vi "SubMatrixVg2.vi"(0 "VgCluster":T1={"Target Voltage, V"=1.0, "Sweep rate, V/min"=1.0, "Time btw \npoints, sec"=1.0, "points at each Vg"=1, "Set compliance limit, mkA"=0.05} {"Set compliance limit, mkA" min=0.0 max=1.0 step=0.01 format="%.3f"; "Time btw \npoints, sec" format="%.2f"; "Sweep rate, V/min" min=0.0 max=1.0 step=0.01 format="%.4f"; "Target Voltage, V" min=-4.0 max=4.0 step=0.1 format="%.4f"}, 1 "Instruments":T3={"Oscillator"=TRUE, "Addr 1 lock-in"=TRUE, "Addr 1 lock-in oop"=TRUE, "Addr 2 lock-in"=FALSE, "Addr 2 lock-in oop"=FALSE, "Addr 3 lock-in"=FALSE, "Addr 3 lock-in oop"=FALSE, "Voltage (Vk1)"=FALSE, "Current (Ik1)"=TRUE, "Voltage (Vk2)"=FALSE, "Current (Ik2)"=FALSE, "Voltage (Vk3)"=FALSE, "Current (Ik3)"=FALSE, "Channel 1 (Vnano1)  "=FALSE, "Channel 2 (Vnano1b)"=FALSE, "Channel 1 (Vnano2)   "=FALSE, "Channel 2 (Vnano2b)"=FALSE, "Thermometer 1 (T1)"=TRUE, "Magnetic Field (B)"=TRUE, "Capacitance (C) and Loss (L)"=FALSE}, 2 "Settings":T2={"Ring 3"=1, "Ring 2"=4, "Fixed Current mkA"=0.5, "If yes, the current is:"=enum."Radio Selection 1", "Ressitance measurements?"=TRUE, "Commute DC current?"=FALSE} {"Ring 3" items=["1 kOhm", "10 kOhm", "100 kOhm", "1 Mohm", "10 mOhm"]; "Ring 2" items=["1 kOhm", "10 kOhm", "100 kOhm", "1 Mohm", "10 MOhm"]}, 3 "Custom Folder":string, 4 "Time Stamp":timestamp) -> ()   [LabVIEW 2017]
uses:
  <vilib>/Utility/file.llb/Write To Spreadsheet File (DBL).vi
panel:
  out "Vk2ini":dbl
  out "Current":dbl
  out "Comments":string[](array[string])
  out "ArrayBoolian":bool[][](array[boolean])
  out "Delib Time delay":i32
  out "XY Graph":cluster{dbl[], dbl[]}(graph)={[1.0, 0.8, 0.6000000000000001, 0.4000000000000001, 0.20000000000000007, 5.551115123125783e-17, -0.19999999999999996, -0.39999999999999997, -0.6, -0.8, -1.0], [0.03352775, 0.056811, 0.03911575, 0.04330675, -0.02468015, 0.011641600000000002, 0.10151450000000001, 0.12386675000000001, 0.08288825000000001, -0.00186266, -0.038650000000000004]}
  out "array for data":dbl[](array[numeric])
  in  "Ring":u16(ring) caption="Y-axis:" items=["Vg"]
  out "Data file:":path
  in  "error in (no error)":errorcluster
  # "Lock-in Amplifiers"
  # "Temperature"
  # "SourceMeters"
  # "Nanovoltmeters"
  # "Main"
  # "(not recommended, too slow)"
  # "Magnetic Field"
  # "Capacitance & Loss"
  # "(not recommended, too slow)"
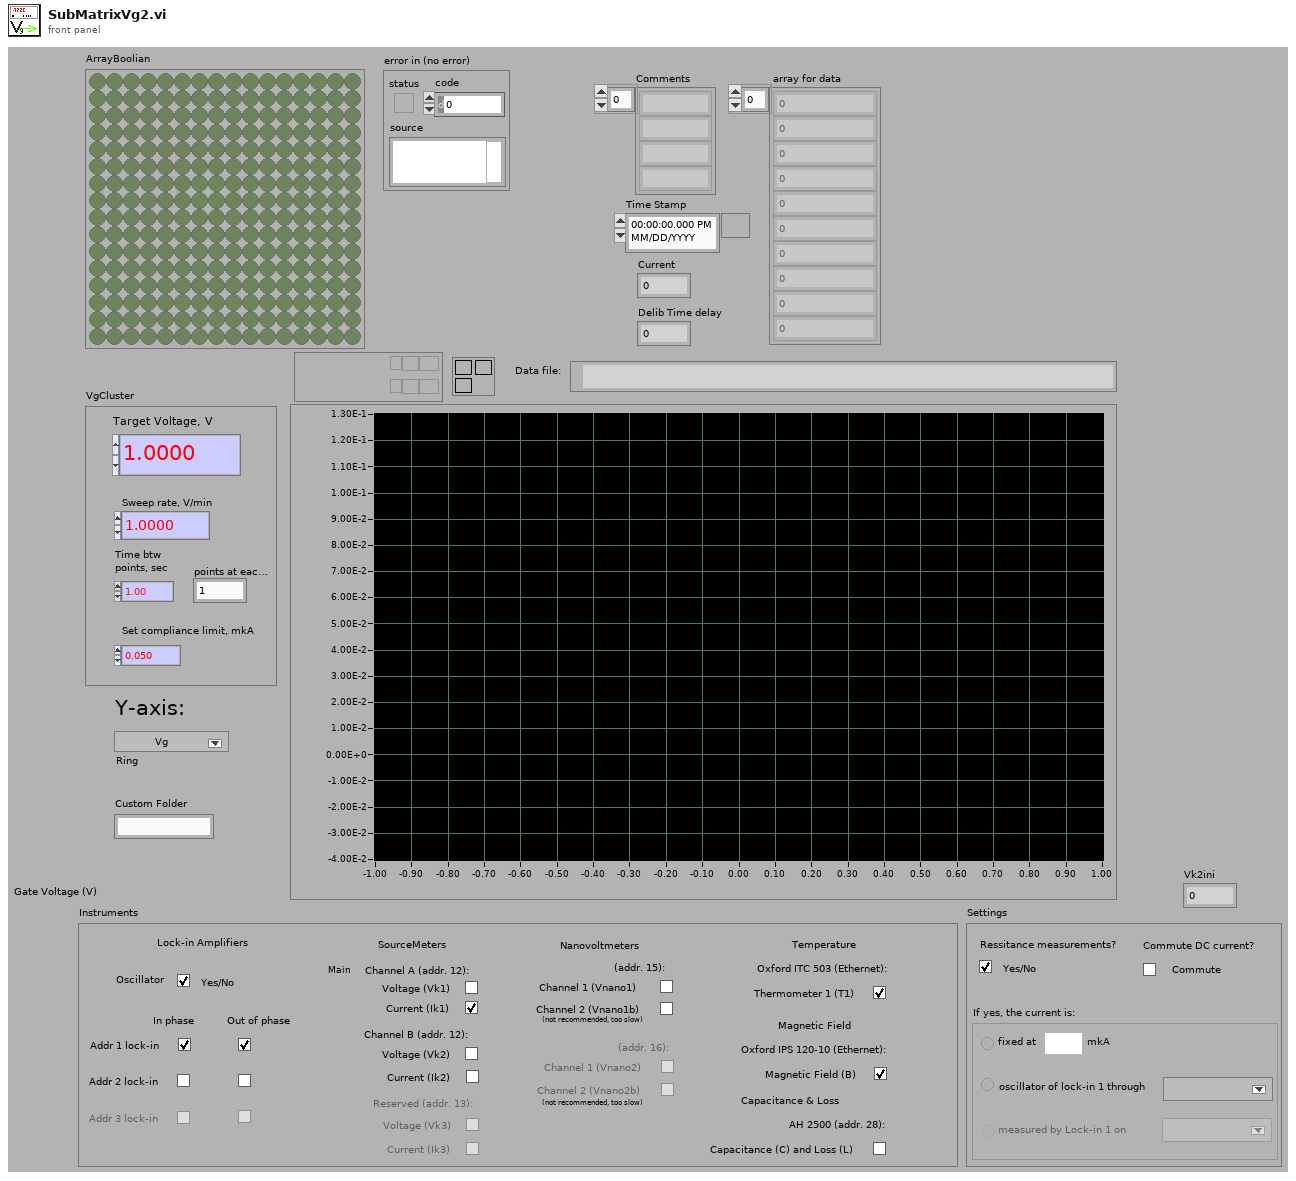
[diagram p1: front panel]
types:
  T1 = cluster{"Target Voltage, V":dbl, "Sweep rate, V/min":dbl, "Time btw \npoints, sec":dbl, "points at each Vg":i32, "Set compliance limit, mkA":dbl}
  T2 = cluster{"Ring 3":u16, "Ring 2":u16, "Fixed Current mkA":dbl, "If yes, the current is:":enum32{"Radio Selection 1", "Radio Selection 2", "Radio Selection 3"}, "Ressitance measurements?":bool, "Commute DC current?":bool}
  T3 = cluster{"Oscillator":bool, "Addr 1 lock-in":bool, "Addr 1 lock-in oop":bool, "Addr 2 lock-in":bool, "Addr 2 lock-in oop":bool, "Addr 3 lock-in":bool, "Addr 3 lock-in oop":bool, "Voltage (Vk1)":bool, "Current (Ik1)":bool, "Voltage (Vk2)":bool, "Current (Ik2)":bool, "Voltage (Vk3)":bool, "Current (Ik3)":bool, "Channel 1 (Vnano1)  ":bool, "Channel 2 (Vnano1b)":bool, "Channel 1 (Vnano2)   ":bool, "Channel 2 (Vnano2b)":bool, "Thermometer 1 (T1)":bool, "Magnetic Field (B)":bool, "Capacitance (C) and Loss (L)":bool}
  T4 = enum32{"Radio Selection 1", "Radio Selection 2", "Radio Selection 3"}
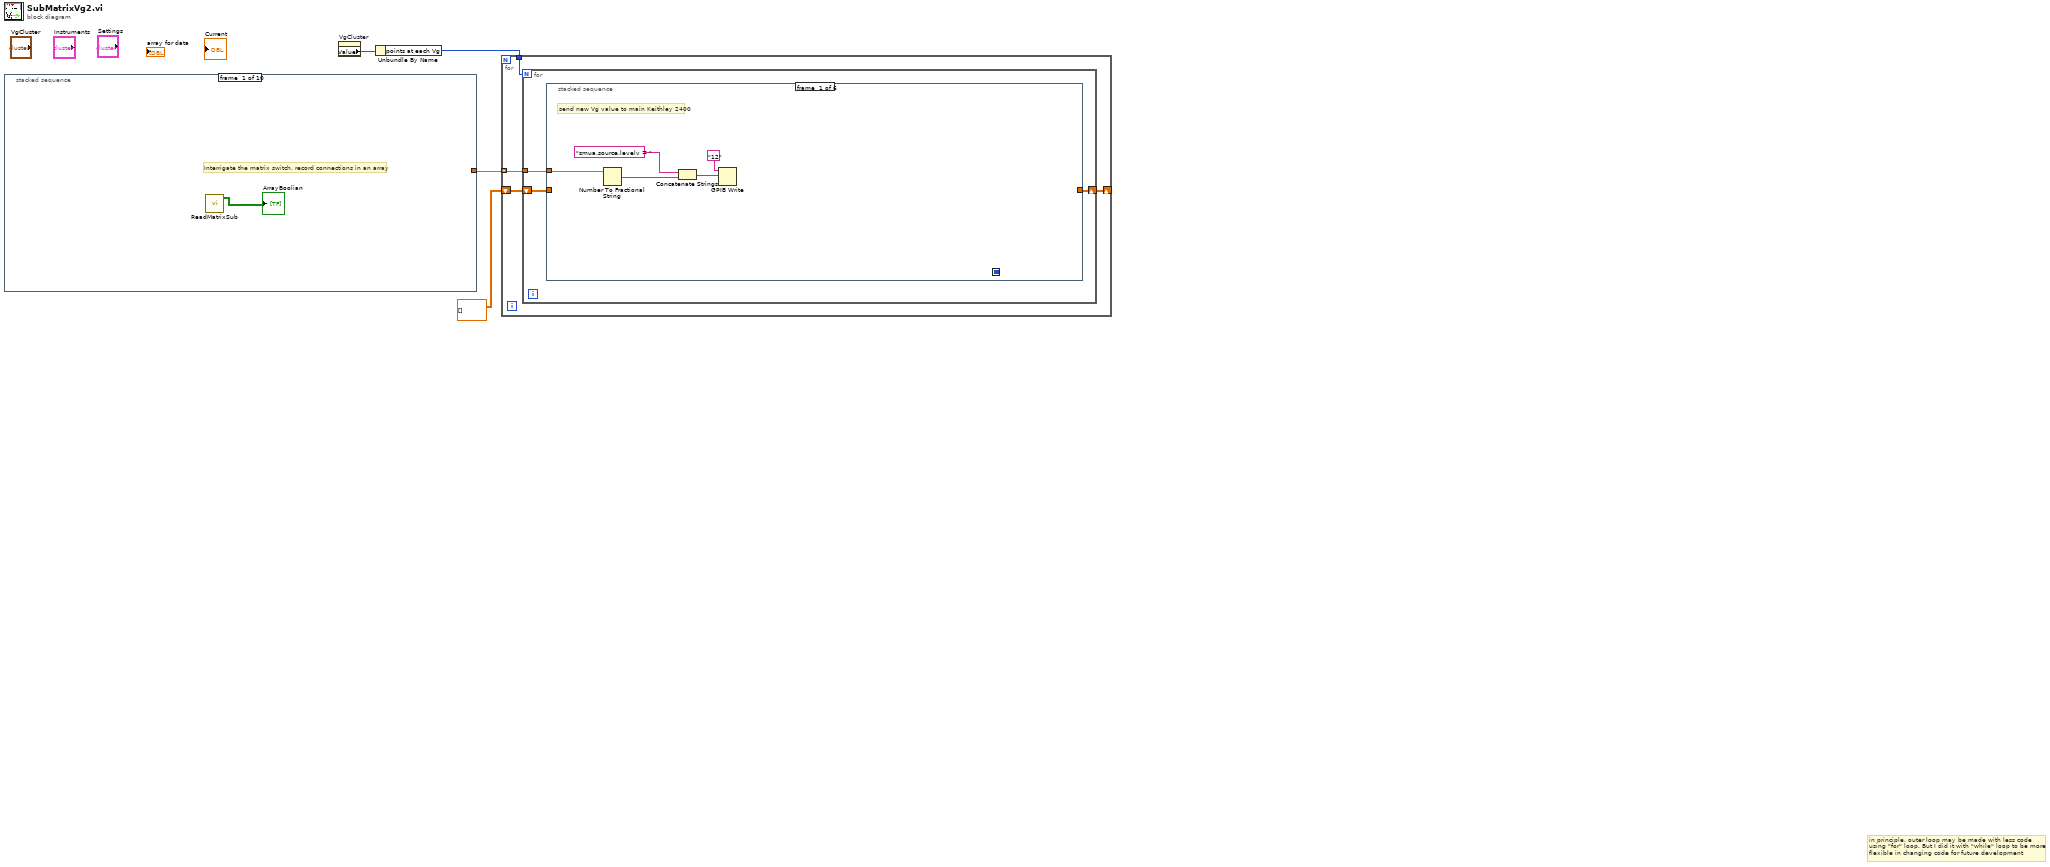
[diagram p0: block diagram]
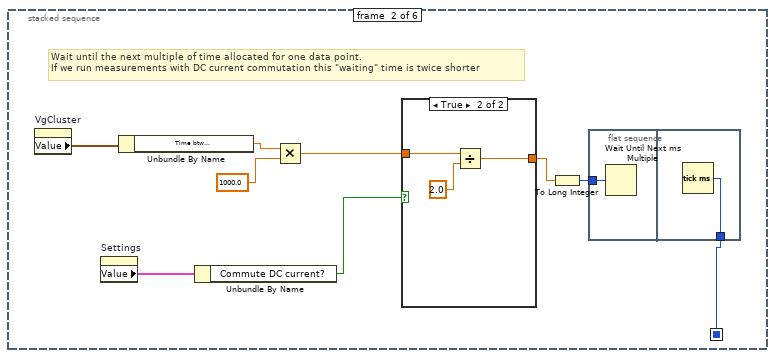
[diagram p2: hidden frame]
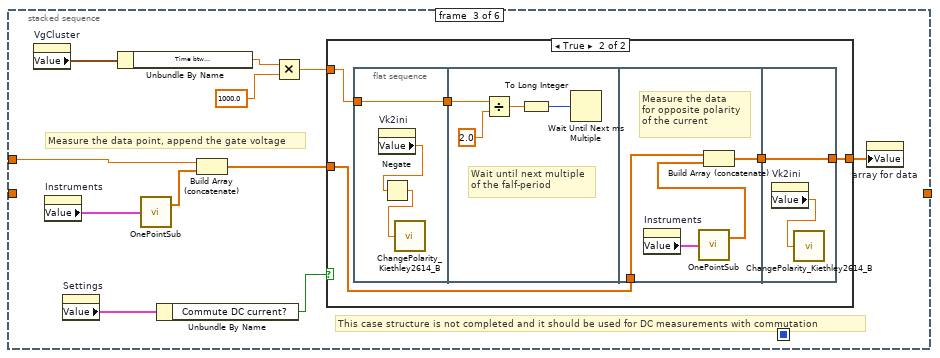
[diagram p4: hidden frame]
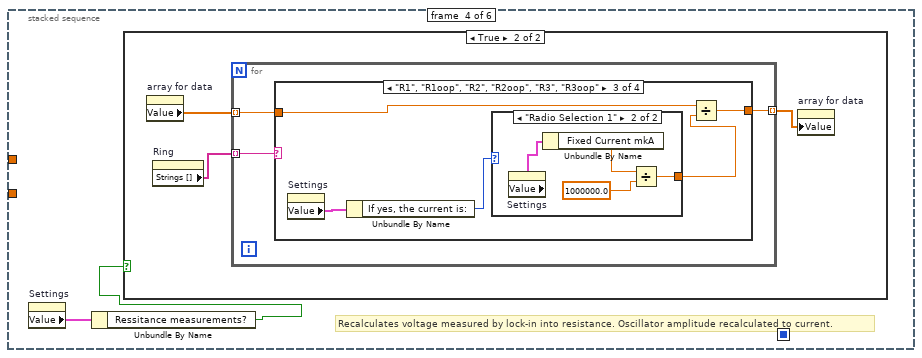
[diagram p6: hidden frame]
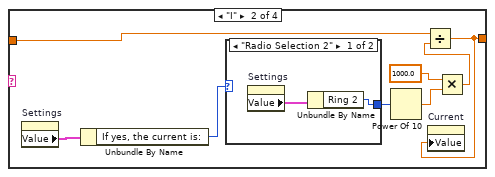
[diagram p9: hidden frame]
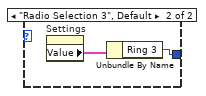
[diagram p10: hidden frame]
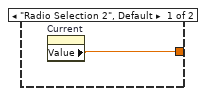
[diagram p11: hidden frame]
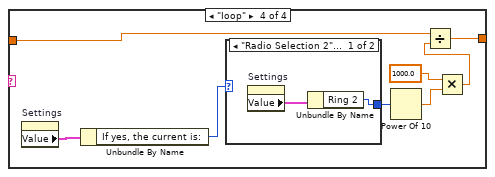
[diagram p12: hidden frame]
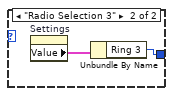
[diagram p13: hidden frame]
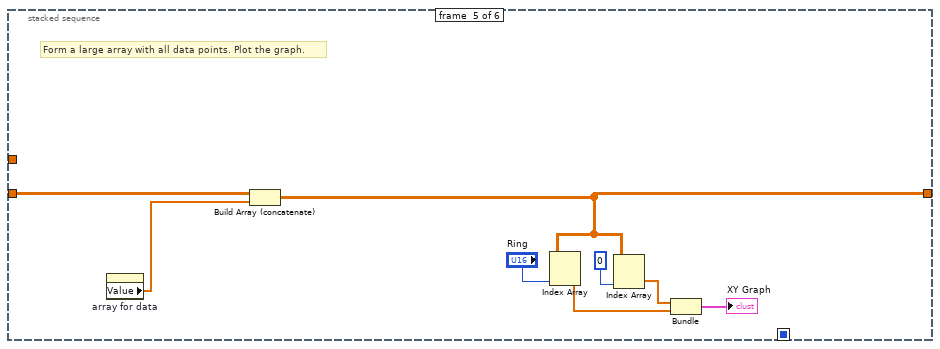
[diagram p14: hidden frame]
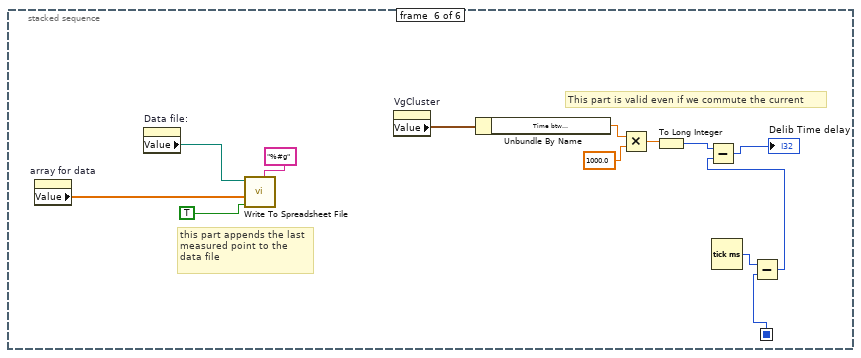
[diagram p15: hidden frame]
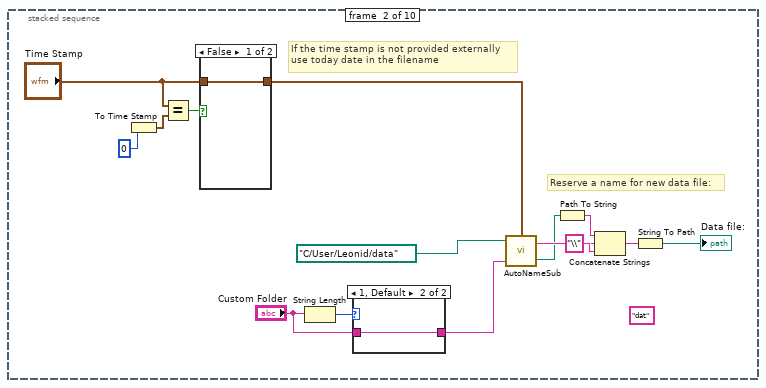
[diagram p16: hidden frame]
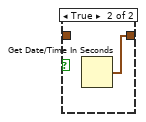
[diagram p17: hidden frame]
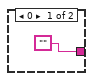
[diagram p18: hidden frame]
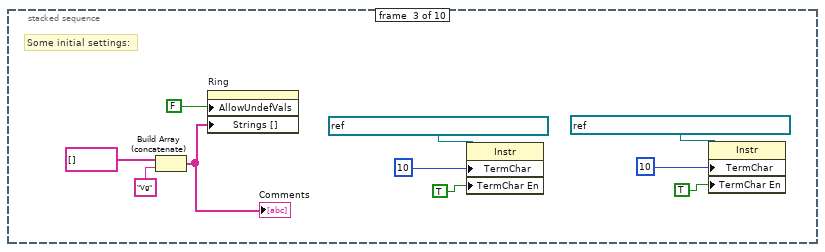
[diagram p19: hidden frame]
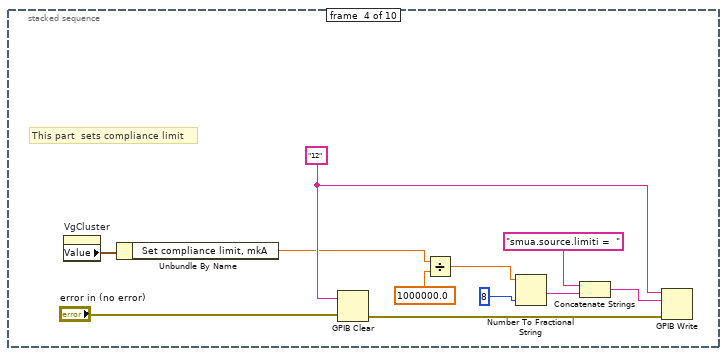
[diagram p20: hidden frame]
diagram:
  # "in principle, outer loop may be made with less code\nusing \"for\" loop. But I did it with \"while\" loop to be more \nflexible in changing code for future development"
  n1 = stacked-sequence {
    tunnel: [_ _ _ _ _ _ _ _ _ w128] -> w4
    frame #0 {
      # "Interrigate the matrix switch, record connections in an array"
      n2 = call "ReadMatrixSub.vi"() -> ("Array"=→"ArrayBoolian":bool[][])  [unwired: 9 in, 2 out]
    }
    frame #1 {
      (unwired) "dat"
      # "If the time stamp is not provided externally\nuse today date in the filename"
      # "Reserve a name for new data file:"
      n3 = To Time Stamp(1:0) -> (0:w9:timestamp)
      n4 = Equal?(x="Time Stamp", y=w9) -> (x = y?=w8:bool)
      n5 = case shown="False" w8 {
        tunnel: "Time Stamp" -> [w21 _]
        tunnel: [w21 w22] -> w6
        frame False {
        }
        frame True {
          n6 = Get Date/Time In Seconds() -> (seconds since 1Jan1904=w22:timestamp)
        }
      }
      n7 = String Length(string="Custom Folder") -> (length=w13:i32)
      n8 = case shown="1, Default" w13 {
        tunnel: "Custom Folder" -> [_ w24]
        tunnel: ["" w24] -> w11
        frame 0 {
        }
        frame 1, Default {
        }
      }
      n9 = call "AutoNameSub.vi"("Time Stamp"=w6, "Custom Folder"=w11, "User Data Folder"=path "C:/User/Leonid/data") -> ("created path"=w19:path, "String"=w20:string)  [unwired: 1 in]
      n10 = Path To String(path=w19) -> (string=w14:string)
      n11 = Concatenate Strings(w14, "\\", w20) -> (w16:string)
      n12 = String To Path(string=w16) -> (path=→"Data file:":path)
    }
    frame #2 {
      # "Some initial settings:"
      n13 = Build Array (concatenate)(string[] [], "Vg") -> (w25:string[])
      "Comments" <- w25
      n14 = property on="Ring" class="Ring (strict)"("AllowUndefVals"=FALSE, "Strings []"=w25) -> ()  [unwired: 2 in, 2 out]
      n15 = property class="Instr"(reference=refnum<visa-resource-name> "TCPIP0::192.168.128.3::7020::SOCKET" ("VISA resource name"), "TermChar"=10, "TermChar En"=TRUE) -> ()  [unwired: 1 in, 2 out]
      n16 = property class="Instr"(reference=refnum<visa-resource-name> "TCPIP0::192.168.128.2::7020::SOCKET" ("VISA resource name"), "TermChar"=10, "TermChar En"=TRUE) -> ()  [unwired: 1 in, 2 out]
    }
    frame #3 {
      w38 = "12"
      # "This part  sets compliance limit"
      n17 = property on="VgCluster" class="Clust (strict)"() -> ("Value"=w36:T1)  [unwired: 2 in, 2 out]
      n18 = Unbundle By Name(w36) -> ("Set compliance limit, mkA"=w35:dbl)
      n19 = GPIB Clear(2:"error in (no error)", 3:w38) -> (0:w39:errorcluster)  [unwired: 1 out]
      n20 = Divide(x=w35, y=1000000.0) -> (x/y=w44:dbl)
      n21 = Number To Fractional String(number=w44, precision (6)=i16 8) -> (F-format string=w41:string)  [unwired: 2 in]
      n22 = Concatenate Strings("smua.source.limiti =  " ("data"), w41) -> (w40:string)
      n23 = GPIB Write(0:w38, 1:w40, 3:w39) -> ()  [unwired: 2 in, 2 out]
    }
    frame #4 {
      # "List of measured parameters obtained as \na text array and \"fed\" to a ring selector"
      # "When current is commutated every data point is measured twice (for both polarities of DC current). Names \nof parameters measured for negative polarity will start with lower case \"c\" (for \"commutated\")"
      # "Measurement of one data point (only to get the names of the parameters to be recorded)"
      n24 = property on="Settings" class="Clust (strict)"() -> ("Value"=w52:T2)  [unwired: 2 in, 2 out]
      n25 = property on="Instruments" class="Clust (strict)"() -> ("Value"=w50:T3)  [unwired: 2 in, 2 out]
      n26 = Unbundle By Name(w52) -> ("Commute DC current?"=w53:bool)
      n27 = call "OnePointSub.vi"("cluster"=w50) -> ("TextArray"=w51:string[], "Array"=w46:dbl[])  [unwired: 2 in]
      n28 = case shown="True" w53 {
        tunnel: w51 -> [w55 w64]
        tunnel: [w57 w64] -> w49
        tunnel: w46 -> [w54 _]
        frame True {
          (unwired) 1
          n29 = for {
            tunnel: w55 -> [w59] mode=indexing
            tunnel: w54 -> [w58] mode=indexing
            n30 = case shown="Default" w59 {
              tunnel: w58 -> [w60 _]
              frame "Vk2" {
                "Vk2ini" <- w60
              }
              frame Default {
              }
            }
          }
          n31 = for {
            tunnel: [w63] -> w56 mode=indexing
            tunnel: w55 -> [w61] mode=indexing
            n32 = Concatenate Strings("c", w61) -> (w63:string)
          }
          n33 = Build Array (concatenate)(w55, w56) -> (w57:string[])
        }
        frame False {
        }
      }
      n34 = Build Array (concatenate)("Vg", w49) -> (w47:string[])
      n35 = property on="Ring" class="Ring (strict)"("Strings []"=w47) -> ()  [unwired: 2 in, 2 out]
    }
    frame #5 {
      # "If resistance is not something that we are interested in, then replace \"R\" with \"V\" in all strings"
      n36 = property on="Settings" class="Clust (strict)"() -> ("Value"=w65:T2)  [unwired: 2 in, 2 out]
      n37 = Unbundle By Name(w65) -> ("Ressitance measurements?"=w66:bool)
      n38 = case shown="False" w66 {
        frame True {
        }
        frame False {
          n39 = property on="Ring" class="Ring (strict)"() -> ("Strings []"=w68:string[])  [unwired: 2 in, 2 out]
          n40 = for {
            tunnel: w68 -> [w71] mode=indexing
            tunnel: [w69] -> w67 mode=indexing
            n41 = String Subset(string=w71, length (rest)=1) -> (substring=w73:string)  [unwired: 1 in]
            n42 = Equal?(x=w73, y="R") -> (x = y?=w72:bool)
            n43 = case shown="True" w72 {
              tunnel: w71 -> [w75 w79]
              tunnel: [w75 w76] -> w69
              frame False {
              }
              frame True {
                n44 = Replace Substring(2:1, 4:"V", 5:w79) -> (1:w76:string)  [unwired: 1 in, 1 out]
              }
            }
          }
          n45 = property on="Ring" class="Ring (strict)"("Strings []"=w67) -> ()  [unwired: 2 in, 2 out]
        }
      }
    }
    frame #6 {
      # "This part makes comment line for the \ndata file. Comments are very useful for\ndouble checking that connections are \ncorrect when the data file is opened\nin Origin."
      # "Check how the oscillator is wired to the matrix switch and record connection as a comment"
      n46 = property on="Instruments" class="Clust (strict)"() -> ("Value"=w82:T3)  [unwired: 2 in, 2 out]
      n47 = property on="Comments" class="Arr (strict)"() -> ("Value"=w81:string[])  [unwired: 2 in, 2 out]
      n48 = Unbundle By Name(w82) -> ("Oscillator"=w83:bool)
      n49 = case shown="True" w83 {
        tunnel: [w84 w87] -> w80
        tunnel: w81 -> [w84 w86]
        frame False {
          # "we are not measuring oscillator from\nlock-in (address 1)"
        }
        frame True {
          (unwired) "I"
          # "This subVI takes the matrix column # (instrument\nconnection point) as an argument and finds the raw\n# (contact) to which the instrument is connected"
          # "we are  measuring oscillator"
          n50 = property on="ArrayBoolian" class="Arr (strict)"() -> ("Value"=w90:bool[][])  [unwired: 2 in, 2 out]
          n51 = GPIB Clear(3:"1") -> ()  [unwired: 1 in, 2 out]
          n52 = call "FindInstrConnect.vi"("Column #"=1, "ArrayBoolian"=w90) -> ("String"=w91:string)  [unwired: 1 in, 2 out]
          n53 = call "FindInstrConnect.vi"("Column #"=0, "ArrayBoolian"=w90) -> ("String"=w88:string)  [unwired: 1 in, 2 out]
          n54 = Concatenate Strings(w88, "-", w91) -> (w85:string)
          n55 = Build Array (concatenate)(w86, w85) -> (w87:string[])
        }
      }
      n56 = property on="Comments" class="Arr (strict)"("Value"=w80) -> ()  [unwired: 2 in, 2 out]
    }
    frame #7 {
      # "Check how the input of Lock-in 1 is wired the the matrix switch and record connection as a comment"
      n57 = property on="Instruments" class="Clust (strict)"() -> ("Value"=w97:T3)  [unwired: 2 in, 2 out]
      n58 = property on="Comments" class="Arr (strict)"() -> ("Value"=w96:string[])  [unwired: 2 in, 2 out]
      n59 = Unbundle By Name(w97) -> ("Addr 1 lock-in"=w98:bool)
      n60 = case shown="True" w98 {
        tunnel: [w99 w102] -> w95
        tunnel: w96 -> [w99 w101]
        frame False {
          # "we are not measuring oscillator from\nlock-in (address 1)"
        }
        frame True {
          (unwired) "I"
          # "This subVI takes the matrix column # (instrument\nconnection point) as an argument and finds the raw\n# (contact) to which the instrument is connected"
          # "we are  measuring Lock-In 1"
          n61 = property on="ArrayBoolian" class="Arr (strict)"() -> ("Value"=w105:bool[][])  [unwired: 2 in, 2 out]
          n62 = GPIB Clear(3:"1") -> ()  [unwired: 1 in, 2 out]
          n63 = call "FindInstrConnect.vi"("Column #"=3, "ArrayBoolian"=w105) -> ("String"=w106:string)  [unwired: 1 in, 2 out]
          n64 = call "FindInstrConnect.vi"("Column #"=2, "ArrayBoolian"=w105) -> ("String"=w103:string)  [unwired: 1 in, 2 out]
          n65 = Concatenate Strings(w103, "-", w106) -> (w100:string)
          n66 = Build Array (concatenate)(w101, w100) -> (w102:string[])
        }
      }
      n67 = property on="Comments" class="Arr (strict)"("Value"=w95) -> ()  [unwired: 2 in, 2 out]
    }
    frame #8 {
      w118 = "\r"
      w117 = "\n"
      # "Both lines are recorded into\nthe data file."
      # "This part converts string array with the names of measured parameters into the line of text separated by TABs. The resulting string is\nrecorded as the first line of the data file. The second line is comments with information about conections of the instruments to particular contacts."
      n68 = property on="Ring" class="Ring (strict)"() -> ("Strings []"=w111:string[])  [unwired: 2 in, 2 out]
      n69 = property on="Comments" class="Arr (strict)"() -> ("Value"=w116:string[])  [unwired: 2 in, 2 out]
      n70 = for {
        tunnel: w111 -> [w126] mode=indexing
        shift-right: [w124] -> w114
        shift-left: "" -> [w125]
        n71 = Concatenate Strings(w125, w126, "\t") -> (w124:string)
      }
      n72 = for {
        tunnel: w116 -> [w122] mode=indexing
        shift-right: [w120] -> w119
        shift-left: "" -> [w121]
        n73 = Concatenate Strings(w121, w122, "\t") -> (w120:string)
      }
      n74 = Concatenate Strings(w114, w118, w117, w118, w117, w119, w118, w117) -> (w112:string)
      n75 = property on="Data file:" class="Path"() -> ("Value"=w110:path)  [unwired: 2 in, 2 out]
      n76 = Write to Text File(file (use dialog)=w110, text=w112) -> ()  [unwired: 2 in, 3 out]
    }
    frame #9 {
      w142 = "12"
      # "Then the table is made with all values\nof the gate voltage to be measured"
      # "rounding to 0.1 V"
      # "This part reads the output voltage on channel A of the main Keithly 2614B \n(address 12)"
      n77 = property on="VgCluster" class="Clust (strict)"() -> ("Value"=w136:T1)  [unwired: 2 in, 2 out]
      n78 = Unbundle By Name(w136) -> ("Target Voltage, V"=w130:dbl, "Sweep rate, V/min"=w135:dbl, "Time btw \npoints, sec"=w134:dbl)
      n79 = GPIB Write(0:w142, 1:"print(smua.measure.v())" ("data")) -> (6:w145:errorcluster)  [unwired: 3 in, 1 out]
      n80 = GPIB Read(0:w142, 1:200 ("byte count"), 3:w145) -> (5:w137:string)  [unwired: 2 in, 2 out]
      n81 = Fract/Exp String To Number(string=w137) -> (number=w141:dbl)  [unwired: 3 in, 1 out]
      n82 = Multiply(x=w135, y=w134) -> (x*y=w133:dbl)
      n83 = Divide(x=w133, y=60.0) -> (x/y=w129:dbl)
      n84 = Number To Fractional String(number=w141, width (-)=5, precision (6)=1) -> (F-format string=w138:string)  [unwired: 1 in]
      n85 = Fract/Exp String To Number(string=w138) -> (number=w131:dbl)  [unwired: 3 in, 1 out]
      n86 = call "LinTableSubVI.vi"("Step"=w129, "Final"=w130, "Initial"=w131) -> ("Array"=w128:dbl[])  [unwired: 1 in]
    }
  }
  n87 = property on="VgCluster" class="Clust (strict)"() -> ("Value"=w3:T1)  [unwired: 2 in, 2 out]
  n88 = Unbundle By Name(w3) -> ("points at each Vg"=w2:i32)
  n89 = for {
    tunnel: w4 -> [w149] mode=indexing
    tunnel: w2 -> [w148]
    shift-right: [w146] -> _
    shift-left: dbl[][] [] -> [w147]
    n90 = for {
      N: w148 -> [_]
      tunnel: w149 -> [w152]
      shift-right: [w150] -> w146
      shift-left: w147 -> [w151]
      n91 = stacked-sequence {
        seq-local: [_ w158 _ _ _ _] -> [_ _ _ _ _ w261]
        tunnel: w152 -> [w154 _ w175 _ _ _]
        tunnel: w151 -> [_ _ _ _ w248 _]
        tunnel: [_ _ _ _ w246 _] -> w150
        frame #0 {
          # "send new Vg value to main Keithley 2400"
          n92 = Number To Fractional String(number=w154) -> (F-format string=w156:string)  [unwired: 3 in]
          n93 = Concatenate Strings("smua.source.levelv = " ("data"), w156) -> (w155:string)
          n94 = GPIB Write(0:"12", 1:w155) -> ()  [unwired: 3 in, 2 out]
        }
        frame #1 {
          # "Wait until the next multiple of time allocated for one data point.\nIf we run measurements with DC current commutation this \"waiting\" time is twice shorter"
          n95 = property on="VgCluster" class="Clust (strict)"() -> ("Value"=w166:T1)  [unwired: 2 in, 2 out]
          n96 = property on="Settings" class="Clust (strict)"() -> ("Value"=w163:T2)  [unwired: 2 in, 2 out]
          n97 = Unbundle By Name(w166) -> ("Time btw \npoints, sec"=w165:dbl)
          n98 = Unbundle By Name(w163) -> ("Commute DC current?"=w162:bool)
          n99 = Multiply(x=w165, y=1000.0) -> (x*y=w161:dbl)
          n100 = case shown="True" w162 {
            tunnel: w161 -> [w169 w171]
            tunnel: [w169 w170] -> w160
            frame False {
            }
            frame True {
              n101 = Divide(x=w171, y=2.0) -> (x/y=w170:dbl)
            }
          }
          n102 = To Long Integer(number=w160) -> (32bit integer=w159:i32)
          n103 = flat-sequence {
            tunnel: w159 -> [w167]
            tunnel: [w168] -> w158
            frame #0 {
              n104 = Wait Until Next ms Multiple(millisecond multiple=w167) -> ()  [unwired: 1 out]
            }
            frame #1 {
              n105 = Tick Count (ms)() -> (millisecond timer value=w168:u32)
            }
          }
        }
        frame #2 {
          # "This case structure is not completed and it should be used for DC measurements with commutation"
          # "Measure the data point, append the gate voltage"
          n106 = property on="VgCluster" class="Clust (strict)"() -> ("Value"=w183:T1)  [unwired: 2 in, 2 out]
          n107 = property on="Instruments" class="Clust (strict)"() -> ("Value"=w177:T3)  [unwired: 2 in, 2 out]
          n108 = property on="Settings" class="Clust (strict)"() -> ("Value"=w180:T2)  [unwired: 2 in, 2 out]
          n109 = Unbundle By Name(w183) -> ("Time btw \npoints, sec"=w182:dbl)
          n110 = call "OnePointSub.vi"("cluster"=w177) -> ("Array"=w176:dbl[])  [unwired: 2 in, 1 out]
          n111 = Unbundle By Name(w180) -> ("Commute DC current?"=w179:bool)
          n112 = Build Array (concatenate)(w175, w176) -> (w174:dbl[])
          n113 = Multiply(x=w182, y=1000.0) -> (x*y=w178:dbl)
          n114 = case shown="True" w179 {
            tunnel: w178 -> [_ w189]
            tunnel: [w184 w186] -> w173
            tunnel: w174 -> [w184 w187]
            frame False {
            }
            frame True {
              n115 = flat-sequence {
                tunnel: w189 -> [w192]
                tunnel: [w192] -> w188
                tunnel: w188 -> [w195]
                tunnel: w187 -> [w198]
                tunnel: [w197] -> w185
                tunnel: [w202] -> w186
                tunnel: w185 -> [w202]
                frame #0 {
                  n116 = property on="Vk2ini" class="DigNum (strict)"() -> ("Value"=w190:dbl)  [unwired: 2 in, 2 out]
                  n117 = Negate(x=w190) -> (-x=w191:dbl)
                  n118 = call "ChangePolarity_Kiethley2614_B.vi"("Voltage (sourse)"=w191) -> ()  [unwired: 1 in]
                }
                frame #1 {
                  # "Wait until next multiple\nof the falf-period"
                  n119 = Divide(x=w195, y=2.0) -> (x/y=w193:dbl)
                  n120 = To Long Integer(number=w193) -> (32bit integer=w194:i32)
                  n121 = Wait Until Next ms Multiple(millisecond multiple=w194) -> ()  [unwired: 1 out]
                }
                frame #2 {
                  # "Measure the data\nfor opposite polarity\nof the current"
                  n122 = property on="Instruments" class="Clust (strict)"() -> ("Value"=w200:T3)  [unwired: 2 in, 2 out]
                  n123 = call "OnePointSub.vi"("cluster"=w200) -> ("Array"=w199:dbl[])  [unwired: 2 in, 1 out]
                  n124 = Build Array (concatenate)(w198, w199) -> (w197:dbl[])
                }
                frame #3 {
                  n125 = property on="Vk2ini" class="DigNum (strict)"() -> ("Value"=w201:dbl)  [unwired: 2 in, 2 out]
                  n126 = call "ChangePolarity_Kiethley2614_B.vi"("Voltage (sourse)"=w201) -> ()  [unwired: 1 in]
                }
              }
            }
          }
          n127 = property on="array for data" class="Arr (strict)"("Value"=w173) -> ()  [unwired: 2 in, 2 out]
        }
        frame #3 {
          # "Recalculates voltage measured by lock-in into resistance. Oscillator amplitude recalculated to current."
          n128 = property on="Settings" class="Clust (strict)"() -> ("Value"=w204:T2)  [unwired: 2 in, 2 out]
          n129 = Unbundle By Name(w204) -> ("Ressitance measurements?"=w203:bool)
          n130 = case shown="True" w203 {
            frame False {
            }
            frame True {
              n131 = property on="array for data" class="Arr (strict)"() -> ("Value"=w206:dbl[])  [unwired: 2 in, 2 out]
              n132 = property on="Ring" class="Ring (strict)"() -> ("Strings []"=w207:string[])  [unwired: 2 in, 2 out]
              n133 = for {
                tunnel: w207 -> [w210] mode=indexing
                tunnel: w206 -> [w209] mode=indexing
                tunnel: [w208] -> w205 mode=indexing
                n134 = case shown="\"R1\", \"R1oop\", \"R2\", \"R2oop\", \"R3\", \"R3oop\"" w210 {
                  tunnel: w209 -> [w211 w214 w226 w236]
                  tunnel: [w211 w212 w225 w235] -> w208
                  frame "False", Default {
                  }
                  frame "I" {
                    n135 = property on="Settings" class="Clust (strict)"() -> ("Value"=w219:T2)  [unwired: 2 in, 2 out]
                    n136 = Unbundle By Name(w219) -> ("If yes, the current is:"=w218:T4)
                    n137 = case shown="\"Radio Selection 2\"" w218 {
                      tunnel: [w220 w222] -> w213
                      frame "Radio Selection 2" {
                        n138 = property on="Settings" class="Clust (strict)"() -> ("Value"=w221:T2)  [unwired: 2 in, 2 out]
                        n139 = Unbundle By Name(w221) -> ("Ring 2"=w220:u16)
                      }
                      frame "Radio Selection 3", Default {
                        n140 = property on="Settings" class="Clust (strict)"() -> ("Value"=w223:T2)  [unwired: 2 in, 2 out]
                        n141 = Unbundle By Name(w223) -> ("Ring 3"=w222:u16)
                      }
                    }
                    n142 = Power Of 10(x=w213) -> (10^x=w217:dbl)
                    n143 = Multiply(x=1000.0, y=w217) -> (x*y=w215:dbl)
                    n144 = Divide(x=w214, y=w215) -> (x/y=w212:dbl)
                    n145 = property on="Current" class="DigNum (strict)"("Value"=w212) -> ()  [unwired: 2 in, 2 out]
                  }
                  frame "R1", "R1oop", "R2", "R2oop", "R3", "R3oop" {
                    n146 = property on="Settings" class="Clust (strict)"() -> ("Value"=w228:T2)  [unwired: 2 in, 2 out]
                    n147 = Unbundle By Name(w228) -> ("If yes, the current is:"=w227:T4)
                    n148 = case shown="\"Radio Selection 1\"" w227 {
                      tunnel: [w229 w232] -> w224
                      frame "Radio Selection 2", Default {
                        n149 = property on="Current" class="DigNum (strict)"() -> ("Value"=w229:dbl)  [unwired: 2 in, 2 out]
                      }
                      frame "Radio Selection 1" {
                        n150 = property on="Settings" class="Clust (strict)"() -> ("Value"=w233:T2)  [unwired: 2 in, 2 out]
                        n151 = Unbundle By Name(w233) -> ("Fixed Current mkA"=w231:dbl)
                        n152 = Divide(x=w231, y=1000000.0) -> (x/y=w232:dbl)
                      }
                    }
                    n153 = Divide(x=w226, y=w224) -> (x/y=w225:dbl)
                  }
                  frame "Ioop" {
                    n154 = property on="Settings" class="Clust (strict)"() -> ("Value"=w241:T2)  [unwired: 2 in, 2 out]
                    n155 = Unbundle By Name(w241) -> ("If yes, the current is:"=w240:T4)
                    n156 = case shown="\"Radio Selection 2\", Default" w240 {
                      tunnel: [w242 w244] -> w234
                      frame "Radio Selection 2", Default {
                        n157 = property on="Settings" class="Clust (strict)"() -> ("Value"=w243:T2)  [unwired: 2 in, 2 out]
                        n158 = Unbundle By Name(w243) -> ("Ring 2"=w242:u16)
                      }
                      frame "Radio Selection 3" {
                        n159 = property on="Settings" class="Clust (strict)"() -> ("Value"=w245:T2)  [unwired: 2 in, 2 out]
                        n160 = Unbundle By Name(w245) -> ("Ring 3"=w244:u16)
                      }
                    }
                    n161 = Power Of 10(x=w234) -> (10^x=w239:dbl)
                    n162 = Multiply(x=1000.0, y=w239) -> (x*y=w237:dbl)
                    n163 = Divide(x=w236, y=w237) -> (x/y=w235:dbl)
                  }
                }
              }
              n164 = property on="array for data" class="Arr (strict)"("Value"=w205) -> ()  [unwired: 2 in, 2 out]
            }
          }
        }
        frame #4 {
          # "Form a large array with all data points. Plot the graph."
          n165 = property on="array for data" class="Arr (strict)"() -> ("Value"=w247:dbl[])  [unwired: 2 in, 2 out]
          n166 = Build Array (concatenate)(w248, w247) -> (w246:dbl[][])
          n167 = Index Array(array=w246, index (col)="Ring") -> (element=w253:dbl[])  [unwired: 1 in]
          n168 = Index Array(array=w246, index (col)=0) -> (element=w251:dbl[])  [unwired: 1 in]
          n169 = Bundle(w251, w253) -> (→"XY Graph":cluster{dbl[], dbl[]})  [unwired: 1 in]
        }
        frame #5 {
          # "This part is valid even if we commute the current"
          # "this part appends the last\nmeasured point to the \ndata file"
          n170 = property on="array for data" class="Arr (strict)"() -> ("Value"=w266:dbl[])  [unwired: 2 in, 2 out]
          n171 = property on="Data file:" class="Path"() -> ("Value"=w264:path)  [unwired: 2 in, 2 out]
          n172 = call-poly <vilib>:"Write To Spreadsheet File.vi"("format (%.3f)"="%#g", "append to file? (new file:F)"=TRUE, "1D data"=w266, "file path (dialog if empty)"=w264) -> ()  [unwired: 4 in, 1 out]
          n173 = property on="VgCluster" class="Clust (strict)"() -> ("Value"=w260:T1)  [unwired: 2 in, 2 out]
          n174 = Unbundle By Name(w260) -> ("Time btw \npoints, sec"=w259:dbl)
          n175 = Multiply(x=w259, y=1000.0) -> (x*y=w257:dbl)
          n176 = To Long Integer(number=w257) -> (32bit integer=w256:i32)
          n177 = Tick Count (ms)() -> (millisecond timer value=w262:u32)
          n178 = Subtract(x=w262, y=w261) -> (x-y=w254:u32)
          n179 = Subtract(x=w256, y=w254) -> (x-y=→"Delib Time delay":u32)
        }
      }
    }
  }
